vi "TB-Initialize Mic Correction.vi"(0 "Exposure parameters":T1={"Low cutoff (kHz)"=0.0, "High cutoff (kHz)"=0.0, "Duration (min)"=0.0, "dB SPL"=0.0, "Waveform"=enum."Noise", "WAVfile"=path "", "refWav"=path "", "use mic correction"=FALSE, "micCorrFile"=path "", "Pistonphone Level (dB SPL)"=0.0, "Sampling rate (Hz)"=0.0, "Buffer length (s)"=0.0, "Stream mic"=FALSE, "Fine adjust"={"Max"=0.0, "Min"=0.0}, "Mic gain"=0.0, "atten"=0.0, "Allow Slack"=FALSE, "max starts"=0, "Freq (kHz)"=8.0, "Tma (s)"=0.0, "Streamed"=[], "Drive"="", "Speaker"="", "Mic"="", "Analysis"={"Method"=enum."Default", "resol (Hz)"=0.0, "nfreq"=0, "signal"=""}}, 7 "Sampling rate (Hz)":dbl, 9 "Npts":i32, 11 "error in (no error)":errorcluster) -> (8 "micCorr":dbl[](array[numeric]), 15 "error out":errorcluster)   [LabVIEW 2020]
uses:
  Typedefs/TB-Parameters.ctl
  Typedefs/TB-Analysis Parameters.ctl
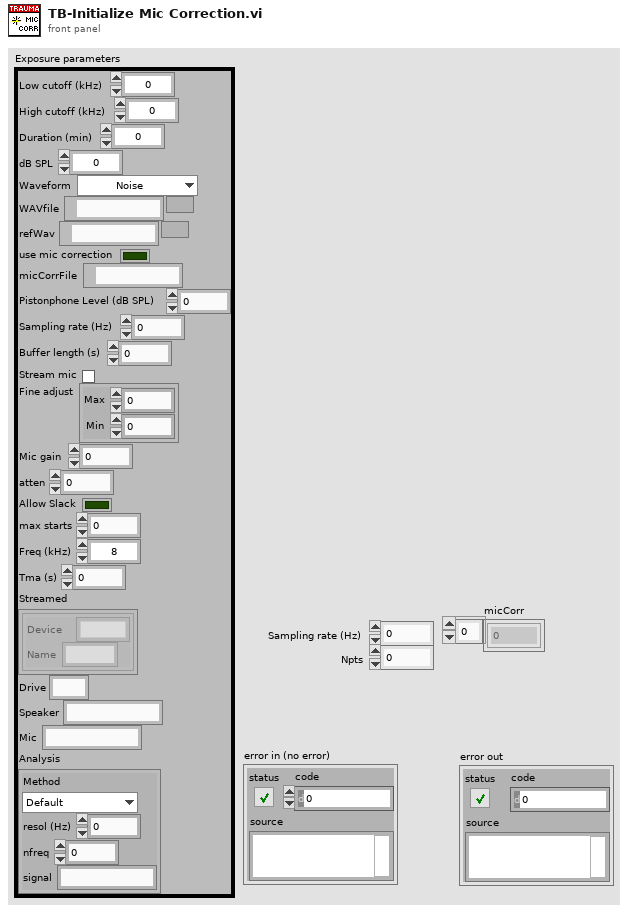
[diagram p1: front panel]
types:
  T1 = typedef "TB-Parameters.ctl" = cluster{"Low cutoff (kHz)":dbl, "High cutoff (kHz)":dbl, "Duration (min)":dbl, "dB SPL":dbl, "Waveform":enum16{"Noise", "File", "Tone"}, "WAVfile":path, "refWav":path, "use mic correction":bool, "micCorrFile":path, "Pistonphone Level (dB SPL)":dbl, "Sampling rate (Hz)":dbl, "Buffer length (s)":dbl, "Stream mic":bool, "Fine adjust":cluster{"Max":dbl, "Min":dbl}, "Mic gain":dbl, "atten":dbl, "Allow Slack":bool, "max starts":i32, "Freq (kHz)":dbl, "Tma (s)":dbl, "Streamed":cluster{"Device":string, "Name":string}[], "Drive":string, "Speaker":string, "Mic":string, "Analysis":T2}
  T2 = typedef "TB-Analysis Parameters.ctl" = cluster{"Method":enum16{"Default", "Periodogram", "Cross-spectrum"}, "resol (Hz)":dbl, "nfreq":i32, "signal":string}
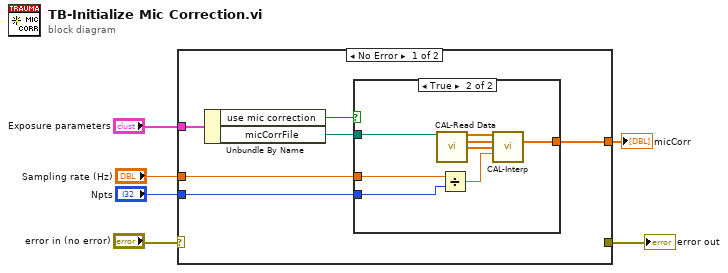
[diagram p0: block diagram]
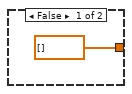
[diagram p2: hidden frame]
diagram:
  n1 = case shown="No Error" "error in (no error)" {
    selector: "error in (no error)" -> [_ w22]
    tunnel: [_ w22] -> w5
    tunnel: "Exposure parameters" -> [w12 _]
    tunnel: "Sampling rate (Hz)" -> [w9 _]
    tunnel: "Npts" -> [w8 _]
    tunnel: [w7 _] -> w1
    frame No Error {
      n2 = Unbundle By Name(w12) -> ("use mic correction"=w11:bool, "micCorrFile"=w10:path)
      n3 = case shown="True" w11 {
        tunnel: w10 -> [_ w21]
        tunnel: w9 -> [_ w16]
        tunnel: w8 -> [_ w15]
        tunnel: [dbl[] [] ("micCorr") w14] -> w7
        frame False {
        }
        frame True {
          n4 = call "CAL-Read Data.vi"("user path"=w21) -> ("Frequency (Hz)"=w20:dbl[], "Mag"=w19:dbl[], "Phase"=w18:dbl[])  [unwired: 10 in, 2 out]
          n5 = Divide(x=w16, y=w15) -> (x/y=w17:dbl)
          n6 = call "CAL-Interp.vi"("Frequency (Hz)"=w20, "Magnitude (dB)"=w19, "Phase (degrees)"=w18, "df (Hz)"=w17) -> ("Interp Magnitude (dB)"=w14:dbl[])  [unwired: 8 in, 3 out]
        }
      }
    }
    frame Error {
    }
  }
  "error out" <- w5
  "micCorr" <- w1
